vi "test file encode.vi"() -> ()   [LabVIEW 2017]
panel:
  out "ascii.ini 2":string
  out "utf8.ini 2":string
  out "utf8.ini":string
  out "ascii.ini":string
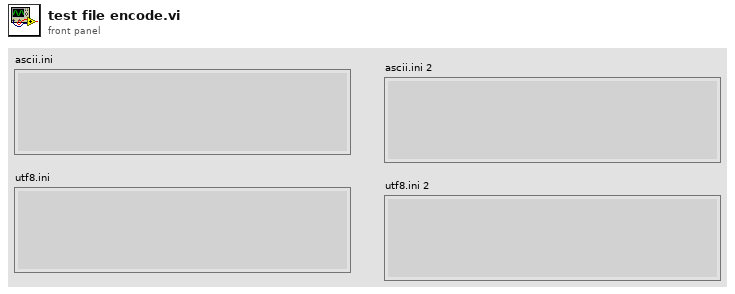
[diagram p1: front panel]
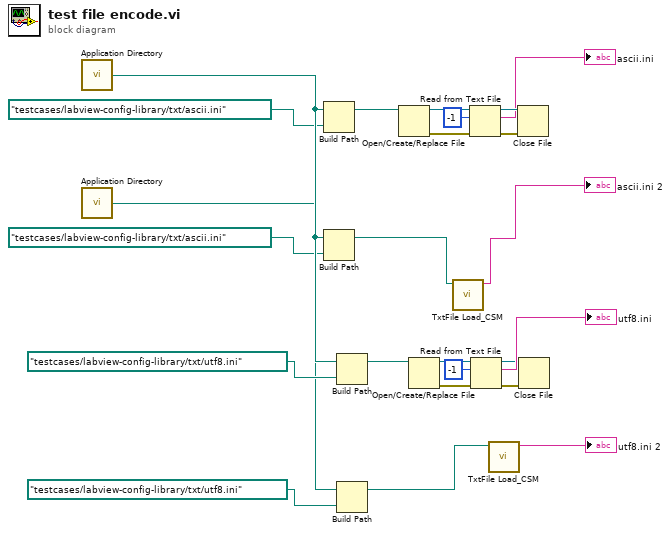
[diagram p0: block diagram]
diagram:
  n1 = call <vilib>:"Application Directory.vi"() -> ("Application Directory"=w9:path)
  n2 = call <vilib>:"Application Directory.vi"() -> ("Application Directory"=w6:path)
  n3 = Build Path(base path=w9, name or relative path=path "testcases/labview-config-library/txt/ascii.ini" ("file path (use dialog)")) -> (appended path=w11:path)
  n4 = Build Path(base path=w6, name or relative path=path "testcases/labview-config-library/txt/ascii.ini" ("file path (use dialog)")) -> (appended path=w2:path)
  n5 = Build Path(base path=w9, name or relative path=path "testcases/labview-config-library/txt/utf8.ini" ("file path (use dialog)")) -> (appended path=w12:path)
  n6 = Build Path(base path=w6, name or relative path=path "testcases/labview-config-library/txt/utf8.ini" ("file path (use dialog)")) -> (appended path=w3:path)
  n7 = Open/Create/Replace File(file path (use dialog)=w11) -> (refnum out=w21:refnum<file>, error out=w22:errorcluster)  [unwired: 5 in, 1 out]
  n8 = Open/Create/Replace File(file path (use dialog)=w12) -> (refnum out=w16:refnum<file>, error out=w15:errorcluster)  [unwired: 5 in, 1 out]
  n9 = call <userlib>:"TxtFile Load_CSM.vi"("Path"=w2) -> ("text"=→"ascii.ini 2":string)  [unwired: 9 in, 1 out]
  n10 = Read from Text File(file (use dialog)=w21, count=-1, error in=w22) -> (refnum out=w23:refnum<file>, text=→"ascii.ini":string, error out=w24:errorcluster)  [unwired: 1 in, 1 out]
  n11 = Read from Text File(file (use dialog)=w16, count=-1, error in=w15) -> (refnum out=w14:refnum<file>, text=→"utf8.ini":string, error out=w13:errorcluster)  [unwired: 1 in, 1 out]
  n12 = call <userlib>:"TxtFile Load_CSM.vi"("Path"=w3) -> ("text"=→"utf8.ini 2":string)  [unwired: 9 in, 1 out]
  n13 = Close File(refnum=w23, error in=w24) -> ()  [unwired: 2 out]
  n14 = Close File(refnum=w14, error in=w13) -> ()  [unwired: 2 out]
